vi "TH_RS232_Init.vi"(4 "error in (no error)":errorcluster, 7 "COMports":refnum<visa-resource-name>[](array[refnum])) -> (0 "error out array":errorcluster[](array[cluster]), 3 "COMhandles":refnum<visa-resource-name>[](array[refnum]))   [LabVIEW 2020]
uses:
  <vilib>/Instr/_visa.llb/VISA Configure Serial Port (Instr).vi
panel:
  in  "timeout (1sec)":u32=1000
  in  "flow control (0:None)":enum16{"None", "XON/XOFF", "RTS/CTS"}(ring)
  in  "stop bits (10: 1 bit)":u16(ring)=10 items=["1.0"=10, "1.5"=15, "2.0"=20]
  in  "parity (0:none)":enum16{"None", "Odd", "Even", "Mark", "Space"}(ring)
  in  "Databits":u32=7
  in  "Baudrate":u32=2400
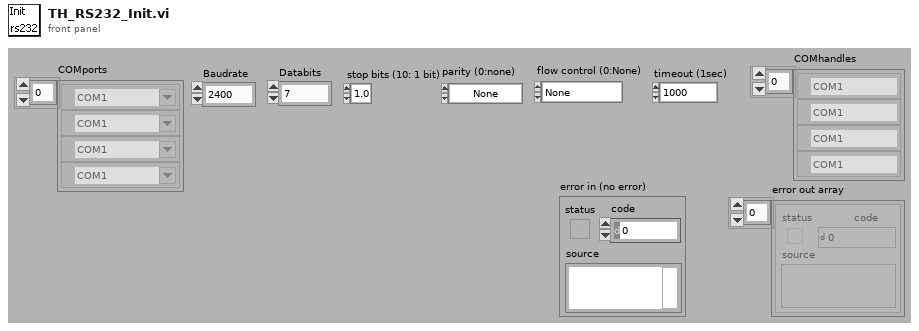
[diagram p1: front panel]
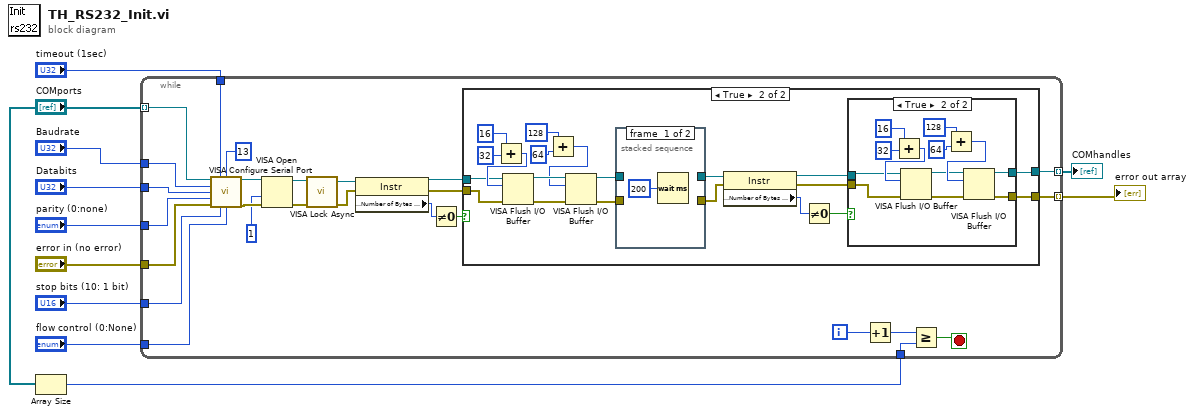
[diagram p0: block diagram]
diagram:
  n1 = Array Size(array="COMports") -> (size(s)=w3:i32)
  n2 = while {
    tunnel: [w19] -> w1 mode=indexing
    tunnel: [w20] -> w2 mode=indexing
    tunnel: w3 -> [w27]
    tunnel: "error in (no error)" -> [w30]
    tunnel: "timeout (1sec)" -> [w32]
    tunnel: "flow control (0:None)" -> [w33]
    tunnel: "stop bits (10: 1 bit)" -> [w34]
    tunnel: "parity (0:none)" -> [w35]
    tunnel: "Databits" -> [w36]
    tunnel: "Baudrate" -> [w37]
    tunnel: "COMports" -> [w29] mode=indexing
    i -> [w28]
    stop <- w25 stop-if-true
    n3 = call-poly "VISA Configure Serial Port"("VISA resource name"=w29, "timeout (10sec)"=w32, "termination char\n(0xA = '\\n' = LF)"=u8 13 ("termination char\n(0xA = '\\n' = LF)"), "baud rate (9600)"=w37, "data bits (8)"=w36, "parity (0:none)"=w35, "error in (no error)"=w30, "stop bits (10: 1 bit)"=w34, "flow control (0:none)"=w33) -> ("VISA resource name out"=w16:refnum<visa-resource-name>, "error out"=w14:errorcluster)  [unwired: 5 in]
    n4 = VISA Open(access mode=u32 1, error in (no error)=w14, VISA resource name=w16) -> (VISA resource name=w15:refnum<visa-resource-name>, error out=w13:errorcluster)  [unwired: 2 in]
    n5 = call <vilib>:"VISA Lock Async.vi"("error in (no error)"=w13, "VISA resource name"=w15) -> ("error out"=w18:errorcluster, "VISA resource name out"=w17:refnum<visa-resource-name>)  [unwired: 7 in, 1 out]
    n6 = property class="Instr"(reference=w17, error in=w18) -> (reference out=w23:refnum<visa-resource-name>, error out=w22:errorcluster, "Serial Settings:Number of Bytes at Serial Port"=w24:u32)
    n7 = Not Equal To 0?(x=w24) -> (x != 0?=w21:bool)
    n8 = case shown="True" w21 {
      tunnel: w23 -> [w39 w51]
      tunnel: w22 -> [w38 w50]
      tunnel: [w39 w41] -> w20
      tunnel: [w38 w40] -> w19
      frame False {
      }
      frame True {
        n9 = Add(x=u16 16 ("mask (16)"), y=u16 32 ("mask (16)")) -> (x+y=w57:u16)
        n10 = VISA Flush I/O Buffer(VISA resource name=w51, mask (16)=w57, error in (no error)=w50) -> (VISA resource name out=w58:refnum<visa-resource-name>, error out=w59:errorcluster)
        n11 = Add(x=u16 128 ("mask (16)"), y=u16 64 ("mask (16)")) -> (x+y=w54:u16)
        n12 = VISA Flush I/O Buffer(VISA resource name=w58, mask (16)=w54, error in (no error)=w59) -> (VISA resource name out=w49:refnum<visa-resource-name>, error out=w48:errorcluster)
        n13 = stacked-sequence {
          tunnel: w49 -> [_ w76]
          tunnel: [_ w76] -> w47
          tunnel: w48 -> [_ w75]
          tunnel: [_ w75] -> w46
          frame #0 {
            n14 = Wait (ms)(milliseconds to wait=u32 200) -> ()  [unwired: 1 out]
          }
          frame #1 {
          }
        }
        n15 = property class="Instr"(reference=w47, error in=w46) -> (reference out=w43:refnum<visa-resource-name>, error out=w42:errorcluster, "Serial Settings:Number of Bytes at Serial Port"=w45:u32)
        n16 = Not Equal To 0?(x=w45) -> (x != 0?=w44:bool)
        n17 = case shown="True" w44 {
          tunnel: w43 -> [w61 w65]
          tunnel: w42 -> [w60 w64]
          tunnel: [w61 w63] -> w41
          tunnel: [w60 w62] -> w40
          frame False {
          }
          frame True {
            n18 = Add(x=u16 16 ("mask (16)"), y=u16 32 ("mask (16)")) -> (x+y=w68:u16)
            n19 = VISA Flush I/O Buffer(VISA resource name=w65, mask (16)=w68, error in (no error)=w64) -> (VISA resource name out=w67:refnum<visa-resource-name>, error out=w66:errorcluster)
            n20 = Add(x=u16 128 ("mask (16)"), y=u16 64 ("mask (16)")) -> (x+y=w71:u16)
            n21 = VISA Flush I/O Buffer(VISA resource name=w67, mask (16)=w71, error in (no error)=w66) -> (VISA resource name out=w63:refnum<visa-resource-name>, error out=w62:errorcluster)
          }
        }
      }
    }
    n22 = Increment(x=w28) -> (x+1=w26:i32)
    n23 = Greater Or Equal?(x=w26, y=w27) -> (x >= y?=w25:bool)
  }
  "COMhandles" <- w2
  "error out array" <- w1
